vi "Serial_Setup_tl.glob.vi"() -> ()   [LabVIEW 2010]
panel:
  in  "Error retries":i32=10
  in  "Timeout retries":i32=10
  in  "Timeout":dbl=0.5 format="%.2f"
  in  "Terminator":string=">"
  in  "flow control etc.":T1={"input XON/XOFF"=FALSE, "input HW Handshake"=FALSE, "input alt HW HShk"=FALSE, "output XON/XOFF"=FALSE, "output HW Handshake"=FALSE, "output alt HW HShk"=FALSE, "XOFF byte "=19, "XON byte"=17, "parity error byte"=0} {"parity error byte" format="%.0x"; "XON byte" format="%.0x"; "XOFF byte" format="%.0x"}
  in  "port number":i32
  in  "buffer size":u16=200
  in  "data bits":u16=8 min=5 max=8 step=1
  in  "parity":u16(ring) items=["no parity", "odd parity", "even parity", "mark parity", "space parity"]
  in  "stop bits":u16(ring) items=["1 bit", "1.5 bits", "2 bits"]
  in  "baud rate":u16=9600
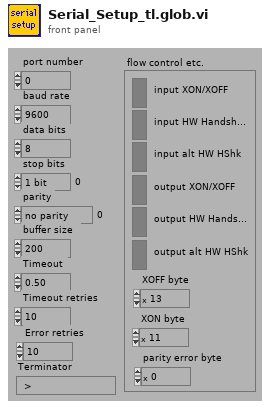
[diagram p1: front panel]
types:
  T1 = cluster{"input XON/XOFF":bool, "input HW Handshake":bool, "input alt HW HShk":bool, "output XON/XOFF":bool, "output HW Handshake":bool, "output alt HW HShk":bool, "XOFF byte ":u8, "XON byte":u8, "parity error byte":u16}
diagram:
